vi "DIAdem Request Report.vi"(0 "Report Path\n(empty - auto PDF in user's folder)":path, 3 "generator settings":T1={"Wait? (t)"=TRUE, "ClientPrint? (f)"=FALSE, "Client (\"\")"="", "joinPDF"=FALSE, "Sort Method"=enum."Template", "Export Row (-1=all)"=-1, "Preview"=FALSE, "Estimate Time"=FALSE, "username"="", "jobid"=""}, 11 "error in (no error)":errorcluster) -> (4 "Output":string, 15 "error out":errorcluster)   [LabVIEW 2011]
uses:
  Datasheet/Datasheet Generator Settings.ctl
  DIAdem Daemon Queue.ctl
  DIAdem Daemon Script Type.ctl
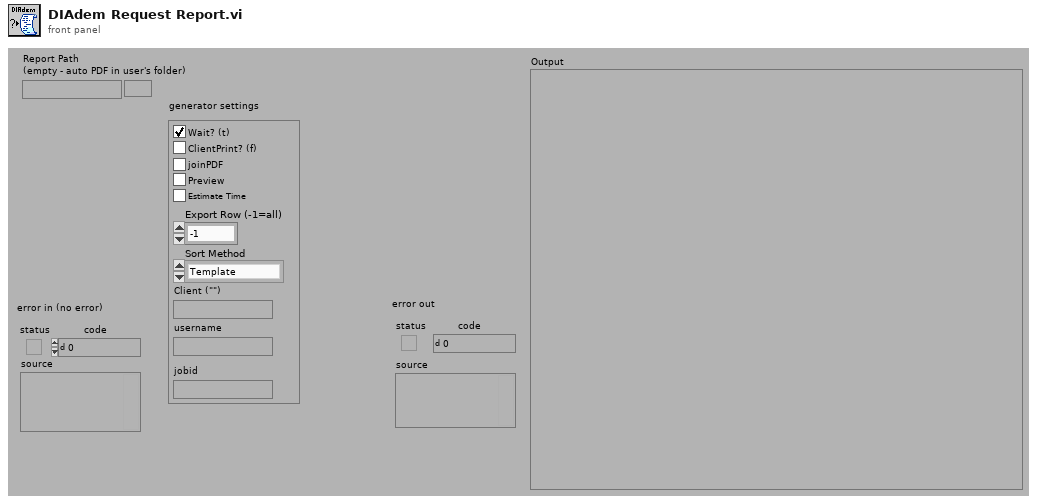
[diagram p1: front panel]
types:
  T1 = typedef "DATASHEET Generator Settings.ctl" = cluster{"Wait? (t)":bool, "ClientPrint? (f)":bool, "Client (\"\")":string, "joinPDF":bool, "Sort Method":enum16{"Item", "Template", "No Sort"}, "Export Row (-1=all)":i32, "Preview":bool, "Estimate Time":bool, "username":string, "jobid":string}
  T2 = typedef "DIAdem Daemon Script Type.ctl" = enum16{"Report", "Query", "Script", "Datasheet", "Append", "Restart", "Stop"}
  T3 = typedef "DIAdem Daemon Queue.ctl" = cluster{"Report Template TDM":path, "Report Processor VBS":path, "Report Path PDF":path, "Report Script Params":string, "Username":string, "Script Type":T2, "Report Query Params":string, "Client Machine":string, "Print on Client?":bool, "Response Queue Name":string, "Script Variables":string[], "Start Request Time":timestamp, "Wait?":bool}
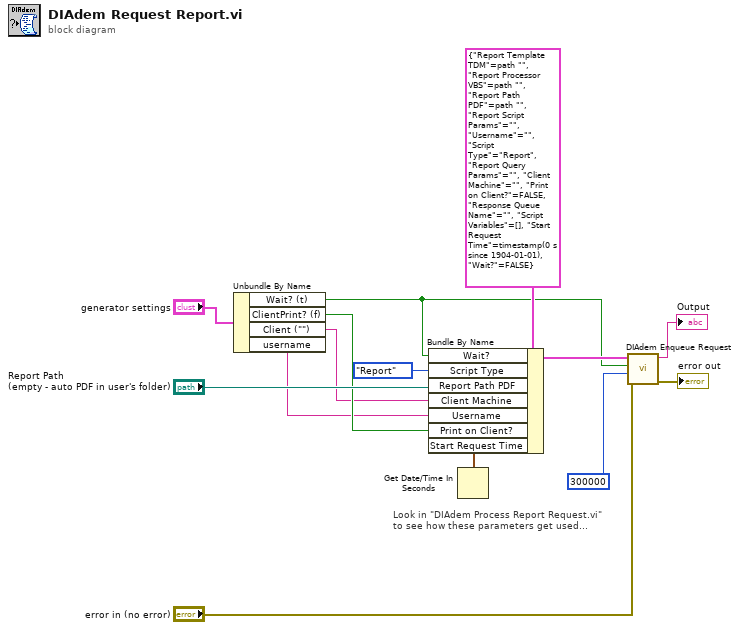
[diagram p0: block diagram]
diagram:
  # "Look in \"DIAdem Process Report Request.vi\"\nto see how these parameters get used..."
  n1 = Unbundle By Name("generator settings") -> ("Wait? (t)"=w1:bool, "ClientPrint? (f)"=w4:bool, "Client (\"\")"=w3:string, "username"=w2:string)
  n2 = Get Date/Time In Seconds() -> (seconds since 1Jan1904=w6:timestamp)
  n3 = Bundle By Name(cluster=T3 {"Report Template TDM"=path "", "Report Processor VBS"=path "", "Report Path PDF"=path "", "Report Script Params"="", "Username"="", "Script Type"=enum."Report", "Report Query Params"="", "Client Machine"="", "Print on Client?"=FALSE, "Response Queue Name"="", "Script Variables"=[], "Start Request Time"=timestamp(0 s since 1904-01-01), "Wait?"=FALSE} ("DD_Report"), "Wait?"=w1, "Script Type"=DIAdem_Daemon_Script_Type."Report", "Report Path PDF"="Report Path\n(empty - auto PDF in user's folder)", "Client Machine"=w3, "Username"=w2, "Print on Client?"=w4, "Start Request Time"=w6) -> (w8:T3)
  n4 = call "DIAdem Enqueue Request.vi"("error in (no error)"="error in (no error)", "timeout in ms (300000)"=300000, "Wait for Completion? (f)"=w1, "DD_Report"=w8) -> ("error out"=→"error out":errorcluster, "Results"=→"Output":string)  [unwired: 6 out]
